vi "Initialize_Power_Meter.vi"(8 "error in (no error)":errorcluster, 11 "VISA Refnum in":refnum<visa-resource-name>="PWR_SENSOR") -> (0 "error out":errorcluster, 3 "VISA resource name out":refnum<visa-resource-name>)   [LabVIEW 2015]
uses:
  <instrlib>/Agilent U2000 Series/Agilent U2000 Series.lvlib
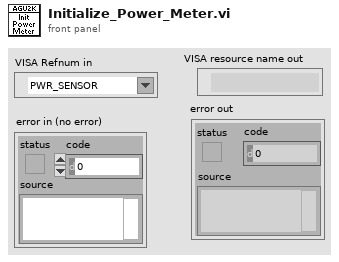
[diagram p1: front panel]
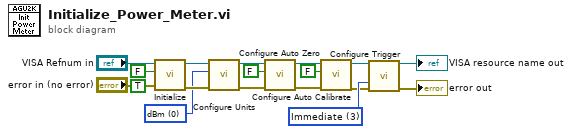
[diagram p0: block diagram]
diagram:
  w12 = u16 0 items=["dBm", "W"] ("Units")
  w17 = 3 items=["Bus", "External", "Hold", "Immediate", "Internal A"] ("Trigger Source (3: Immediate)")
  n1 = call <instrlib>:"Initialize.vi"("error in (no error)"="error in (no error)", "Reset (True)"=TRUE, "ID Query (True)"=FALSE, "VISA resource name"="VISA Refnum in") -> ("error out"=w13:errorcluster, "VISA resource name out"=w14:refnum<visa-resource-name>)  [unwired: 6 out]
  n2 = call <instrlib>:"Configure Units.vi"("error in (no error)"=w13, "Units (0: dBm)"=w12, "VISA resource name"=w14) -> ("error out"=w11:errorcluster, "VISA resource name out"=w10:refnum<visa-resource-name>)  [unwired: 1 in, 6 out]
  n3 = call <instrlib>:"Configure Auto Zero.vi"("error in (no error)"=w11, "Auto Zero (T: Enable)"=FALSE, "VISA resource name"=w10) -> ("error out"=w8:errorcluster, "VISA resource name out"=w7:refnum<visa-resource-name>)  [unwired: 7 in]
  n4 = call <instrlib>:"Configure Auto Calibrate.vi"("error in (no error)"=w8, "Auto Calibrate (T: Enable)"=FALSE, "VISA resource name"=w7) -> ("error out"=w16:errorcluster, "VISA resource name out"=w15:refnum<visa-resource-name>)  [unwired: 7 in]
  n5 = call <instrlib>:"Configure Trigger.vi"("VISA resource name"=w15, "Trigger Source (3: Immediate)"=w17, "error in (no error)"=w16) -> ("VISA resource name out"=→"VISA resource name out":refnum<visa-resource-name>, "error out"=→"error out":errorcluster)  [unwired: 11 in]
